vi "displayChannelList.vi"(8 "error in (no error)":errorcluster, 11 "ActionEditor in":refnum<class "ActionEditor.lvclass">) -> (0 "error out":errorcluster, 3 "ActionEditor out":refnum<class "ActionEditor.lvclass">)   [LabVIEW 2009, in "Views.lvlib" / "ScriptEditor.lvlib" / "ActionEditor.lvclass"]
uses:
  ActionEditor.lvclass
  ActionEditor.lvclass/ActionEditor.ctl
  Tools/Scripting/ScriptingEvent/ScriptEvent.lvclass
  Tools/DatabaseHelpers/Database Objects/ChannelArray/ChannelArray.lvclass
  Tools/DatabaseHelpers/Database Objects/Channel/Channel.lvclass
  Tools/DatabaseHelpers/DbConnection/DeviceDataBase/deviceDataBase.lvclass
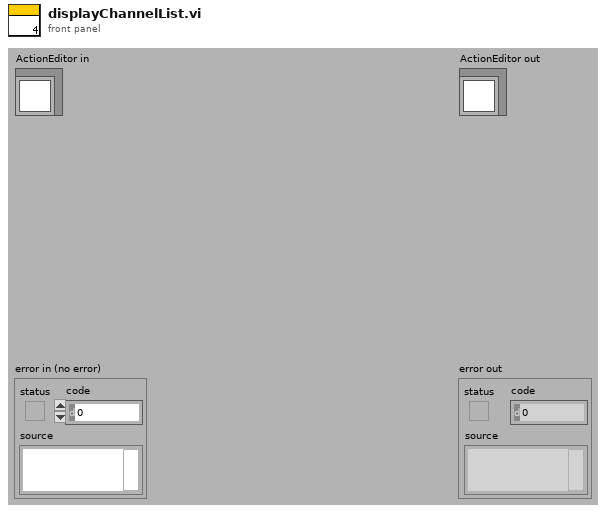
[diagram p1: front panel]
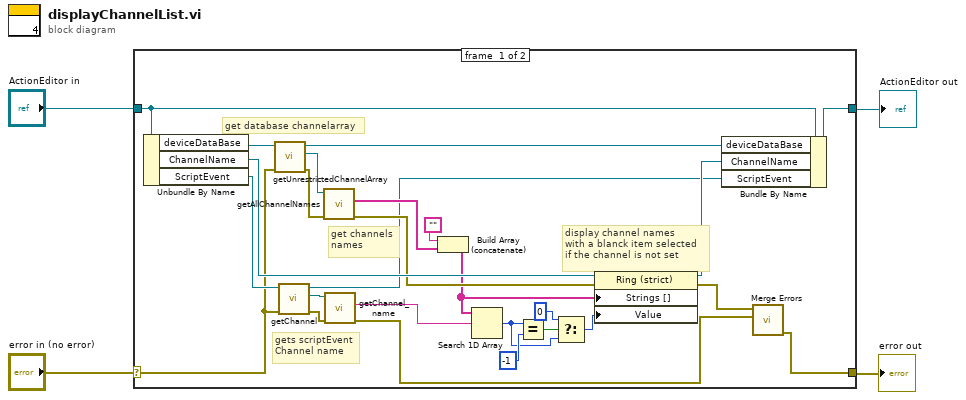
[diagram p0: block diagram]
diagram:
  n1 = case shown="No Error" "error in (no error)" {
    selector: "error in (no error)" -> [w8 w32]
    tunnel: [w11 w32] -> w3
    tunnel: [w26 w31] -> w1
    tunnel: "ActionEditor in" -> [w27 w31]
    frame #0 {
      # "gets scriptEvent\nChannel name"
      # "display channel names\nwith a blanck item selected\nif the channel is not set"
      # "get database channelarray"
      # "get channels\nnames"
      n2 = Unbundle By Name(w27) -> ("deviceDataBase"=w9:refnum<class "deviceDataBase.lvclass">, "ChannelName"=w30:refnum<vi>, "ScriptEvent"=w23:refnum<class "ScriptEvent.lvclass">)
      n3 = call "getUnrestrictedChannelArray.vi"("error in (no error)"=w8, "deviceDataBase in"=w9) -> ("error out"=w6:errorcluster, "ChannelArray.lvclass"=w7:refnum<class "ChannelArray.lvclass">, "deviceDataBase out"=w5:refnum<class "deviceDataBase.lvclass">)  [unwired: 7 in]
      n4 = call-dynamic "getChannel.vi"("error in (no error)"=w8, "ScriptEvent.lvclass in"=w23) -> ("error out"=w21:errorcluster, "Channel.lvclass"=w22:refnum<class "Channel.lvclass">, "ScriptEvent.lvclass out"=w10:refnum<class "ScriptEvent.lvclass">)  [unwired: 7 in]
      n5 = call "getAllChannelNames.vi"("error in (no error)"=w6, "ChannelArray in"=w7) -> ("error out"=w29:errorcluster, "channelNames"=w25:string[])  [unwired: 7 in, 1 out]
      n6 = call "getChannel_name.vi"("error in (no error)"=w21, "Channel.lvclass in"=w22) -> ("error out"=w12:errorcluster, "channel_name"=w19:string)  [unwired: 7 in, 1 out]
      n7 = Build Array (concatenate)("", w25) -> (w20:string[])
      n8 = Search 1D Array(1D array=w20, element=w19) -> (index of element=w15:i32)  [unwired: 1 in]
      n9 = Equal?(x=w15, y=-1) -> (x = y?=w17:bool)
      n10 = Select(t=0, s=w17, f=w15) -> (s? t:f=w14:i32)
      n11 = property class="Ring (strict)"(reference=w30, error in=w29, "Strings []"=w20, "Value"=w14) -> (reference out=w28:refnum<vi>, error out=w13:errorcluster)
      n12 = Bundle By Name(cluster=w27, "deviceDataBase"=w5, "ChannelName"=w28, "ScriptEvent"=w10) -> (w26:refnum<class "ActionEditor.lvclass">)
      n13 = call <vilib>:"Merge Errors.vi"("error in 2 (no error)"=w12, "error in 1 (no error)"=w13) -> ("error out"=w11:errorcluster)  [unwired: 5 in]
    }
    frame #1 {
    }
  }
  "error out" <- w3
  "ActionEditor out" <- w1
